vi "Draw Data1D on Graph ref.vi"(8 "error in (no error)":errorcluster, 10 "Graph ref in":refnum<vi>, 11 "Data1D in":refnum<class "Data1D.lvclass">) -> (0 "error out":errorcluster, 2 "Graph ref out":refnum<vi>, 3 "Data1D out":refnum<class "Data1D.lvclass">)   [LabVIEW 2014, in "Data1D.lvclass"]
uses:
  Data1D.lvclass
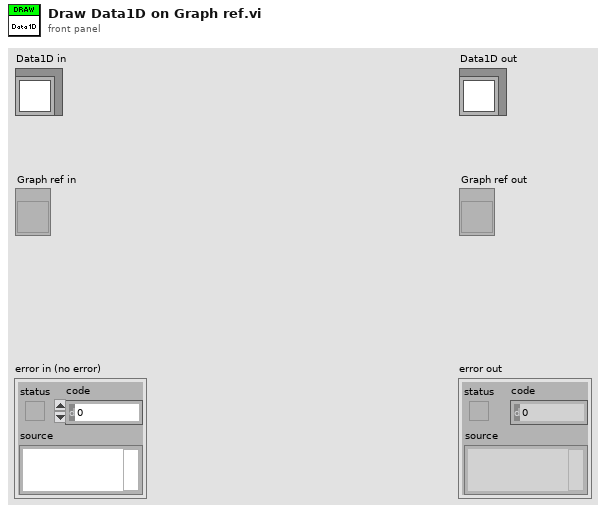
[diagram p1: front panel]
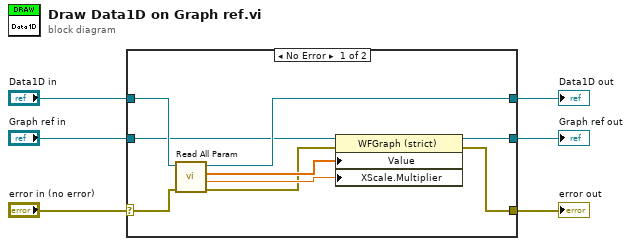
[diagram p0: block diagram]
diagram:
  n1 = case shown="No Error" "error in (no error)" {
    selector: "error in (no error)" -> [w8 w18]
    tunnel: [w14 w18] -> w5
    tunnel: [w10 w17] -> w3
    tunnel: "Data1D in" -> [w11 w17]
    tunnel: "Graph ref in" -> [w7 w16]
    tunnel: [w15 w16] -> w1
    frame No Error {
      n2 = call "Read All Param.vi"("error in (no error)"=w8, "Data1D in"=w11) -> ("error out"=w9:errorcluster, "dt"=w13:dbl, "1D Array"=w12:dbl[], "Data1D out"=w10:refnum<class "Data1D.lvclass">)  [unwired: 5 in, 1 out]
      n3 = property class="WFGraph (strict)"(reference=w7, error in=w9, "Value"=w12, "XScale.Multiplier"=w13) -> (reference out=w15:refnum<vi>, error out=w14:errorcluster)
    }
    frame Error {
    }
  }
  "error out" <- w5
  "Data1D out" <- w3
  "Graph ref out" <- w1
